vi "Channel to Bitmask.vi"(11 "Channel":T1) -> (3 "Numeric":u8)   [LabVIEW 2020, in "MCP23017.lvclass"]
uses:
  MCP23017.lvclass
  GPIO Channel.ctl
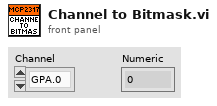
[diagram p1: front panel]
types:
  T1 = typedef "MCP23017.lvclass/GPIO Channel.ctl" = enum16{"GPA.0", "GPA.1", "GPA.2", "GPA.3", "GPA.4", "GPA.5", "GPA.6", "GPA.7", "GPB.0", "GPB.1", "GPB.2", "GPB.3", "GPB.4", "GPB.5", "GPB.6", "GPB.7"}
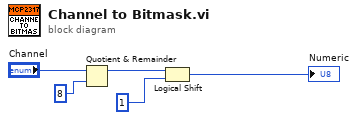
[diagram p0: block diagram]
diagram:
  n1 = Quotient & Remainder(x="Channel", y=8) -> (x-y*floor(x/y)=w3:i32)  [unwired: 1 out]
  n2 = Logical Shift(y=w3, x=u8 1) -> (x << y=→"Numeric":u8)
